vi "ExportToXMI.vi"(0 "reference":refnum<class "ClassDiagramGraph.lvclass">, 1 "nodeInfo":T2, 2 "edgeInfo":T1, 3 "DiagramData":string, 5 "error in (no error)":errorcluster) -> (14 "reference out":refnum<class "ClassDiagramGraph.lvclass">, 16 "XMIText":string, 19 "error out":errorcluster)   [LabVIEW 2016, in "ClassDiagramGraph.lvclass"]
uses:
  <resource>/Framework/Providers/Open_GDS/UML/ClassDiagramGraph_class/ClassDiagramGraph.lvclass
  C:/Program Files (x86)/National Instruments/LabVIEW 2016/resource/Framework/Providers/Open_GDS/UML/Graph_class/Graph.lvclass
  <resource>/Framework/Providers/Open_GDS/ClassProviders/Common/CommonVIs/CommonVIs_ClassNamePathType.ctl
  <resource>/Framework/Providers/Open_GDS/ClassProviders/Common/CommonVIs/CommonVIs_AttributeType.ctl
  <resource>/Framework/Providers/Open_GDS/ClassProviders/Common/CommonVIs/CommonVIs_AttributeDataType.ctl
  <resource>/Framework/Providers/Open_GDS/ClassProviders/Common/String/GDSString_AccessScopeModifierType.ctl
  <resource>/Framework/Providers/Open_GDS/UML/ClassRelationshipEdge_class/private/AssociationType.ctl
  <resource>/Framework/Providers/Open_GDS/UML/General/Point/Point Point2D.ctl
  <resource>/Framework/Providers/Open_GDS/UML/LineStyle_class/LineStyleType.ctl
  <resource>/Framework/Providers/Open_GDS/UML/ArrowHead_class/ArrowHeadType.ctl
  <resource>/Framework/Providers/Open_GDS/UML/PackageNode_class/PackageNode.lvclass
  <resource>/Framework/Providers/Open_GDS/UML/ClassNode_class/ClassNode.lvclass
  <resource>/Framework/Providers/Open_GDS/UML/ArrowHead_class/ArrowHead.lvclass
  <resource>/Framework/Providers/Open_GDS/UML/ClassRelationshipEdge_class/ClassRelationshipEdge.lvclass
  <resource>/Framework/Providers/Open_GDS/UML/LineStyle_class/LineStyle.lvclass
  <resource>/Framework/Providers/Open_GDS/UML/Graph_class/Graph.lvclass
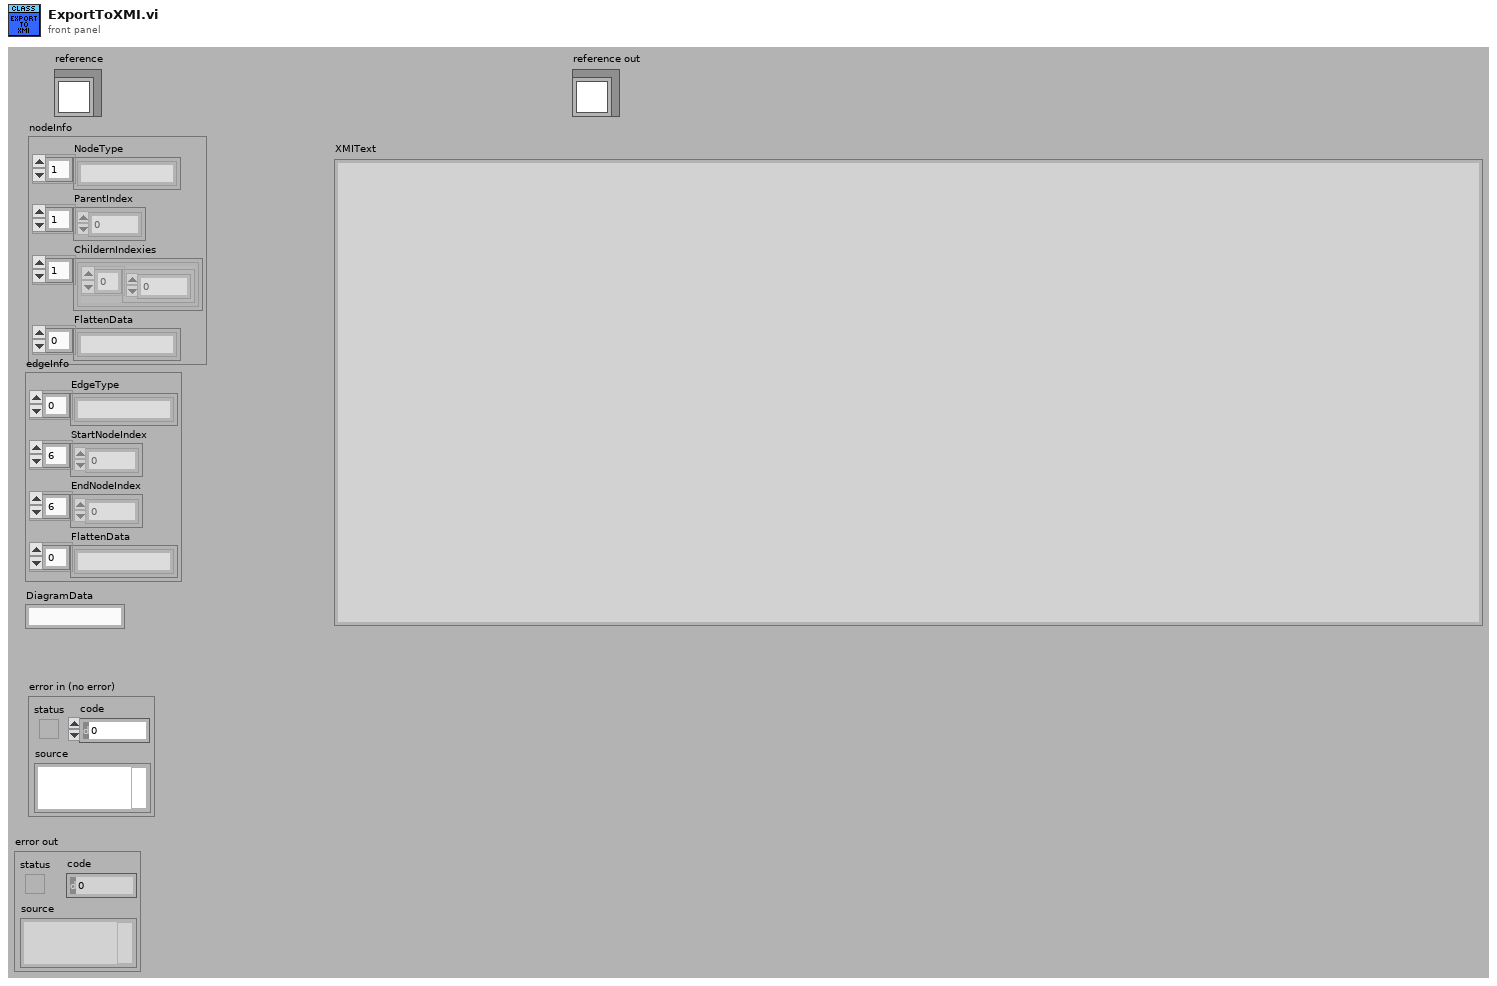
[diagram p1: front panel]
types:
  T1 = cluster{"EdgeType":string[], "StartNodeIndex":i32[], "EndNodeIndex":i32[], "FlattenData":string[]}
  T2 = cluster{"NodeType":string[], "ParentIndex":i32[], "ChildernIndexies":cluster{i32[]}[], "FlattenData":string[]}
  T3 = typedef "CommonVIs_ClassNamePathType.ctl" = cluster{"ClassNamn":string, "ClassPath":path, "InterfaceClass":bool}
  T4 = typedef "CommonVIs_AttributeType.ctl" = cluster{"Name":string, "DataType":T5, "ArrayDim":i32, "CtrlPath":path, "DataTypeString":string, "AccessScope":T6, "InitialData":variant}
  T5 = typedef "CommonVIs_AttributeDataType.ctl" = enum16{"UINT8", "INT8", "UINT16", "INT16", "UINT32", "INT32", "UINT64", "INT64", "SGL", "DBL", "EXT", "CSG", "CDB", "CXT", "TimeStamp", "STRING", "PATH", "BOOL", "ENUM", "RefNum", "VIRefNum", "LabVIEW Class", "Cluster", "Variant", "TypeDef", "Waveform", "LabVIEW Object", "Other", "void"}
  T6 = typedef "GDSString_AccessScopeModifierType.ctl" = enum16{"public", "private", "protected", "internal"}
  T7 = typedef "ClassRelationshipEdge.lvclass/AssociationType.ctl" = u16
  T8 = cluster{"NodeNames":string[], "Attributes":cluster{"attributes":string[]}[], "Methods":cluster{"attributes":string[]}[], "StereoType":string[], "ClassInfo":T3[], "ClassAttributes":cluster{"Attributes":T4[]}[], "RelationShipTypes":T7[], "DataTypes":T5[], "NodeTypes":enum16{"Class", "NotSpecified", "Package", "Note", "Interface"}[], "Text":string, "NodeRelationships":cluster{cluster{"index of element":i32, "RelationType":T7}[]}[], "Ass":cluster{string, i32, "index of element":i32}[]}
  T9 = typedef "Point Point2D.ctl" = cluster{"x":dbl, "y":dbl}
  T10 = cluster{"Attributes":cluster{"Base class":cluster{"Base class":cluster{"Base class":cluster{"start":refnum<k1>, "end":refnum<k1>}}, "lineStyle":refnum<k1>, "startArrowHead":refnum<k1>, "endArrowHead":refnum<k1>, "startLabel":string, "midLabel":string, "endLabel":string, "MidLabelOffset":T9, "SplitWire":bool}, "bentStyleRef":refnum<k1>, "startConnectionOffset":cluster{"x":i32, "y":i32}, "endConnectionOffset":cluster{"x":i32, "y":i32}, "MidLineOffset":cluster{"x":i32, "y":i32}, "DepClass":cluster{"ThisVIs/Ctls":path[], "Dependent_VIs/Ctls":path[]}}, string, string, string, string}
  T11 = typedef "ArrowHead.lvclass/ArrowHeadType.ctl" = enum16{"NONE", "TRIANGLE", "BLACK_TRIANGLE", "V", "HALF_V", "DIAMOND", "BLACK_DIAMOND"}
  T12 = typedef "LineStyle.lvclass/LineStyleType.ctl" = enum16{"SOLID", "DOTTED"}
  T13 = cluster{"index of element":i32, "RelationType":T7}[]
  T14 = enum16{"Class", "NotSpecified", "Package", "Note", "Interface"}
  T15 = typedef "Graph.lvclass/ObjectAttributes.ctl" = cluster{"nodes":refnum<class "AbstractNode.lvclass">[], "edges":refnum<class "AbstractEdge.lvclass">[], "nodesToBeRemoved":refnum<class "AbstractNode.lvclass">[], "edgesToBeRemoved":refnum<class "AbstractEdge.lvclass">[], "needsLayout":bool, "LayoutNodes":refnum<class "AbstractNode.lvclass">[]}
  T16 = cluster{"index of element":i32, "RelationType":T7}
  T17 = cluster{cluster{"index of element":i32, "RelationType":T7}[]}
  T18 = enum16{"Class", "NotSpecified", "Package", "Note", "Interface"}[]
  T19 = cluster{cluster{"index of element":i32, "RelationType":T7}[]}[]
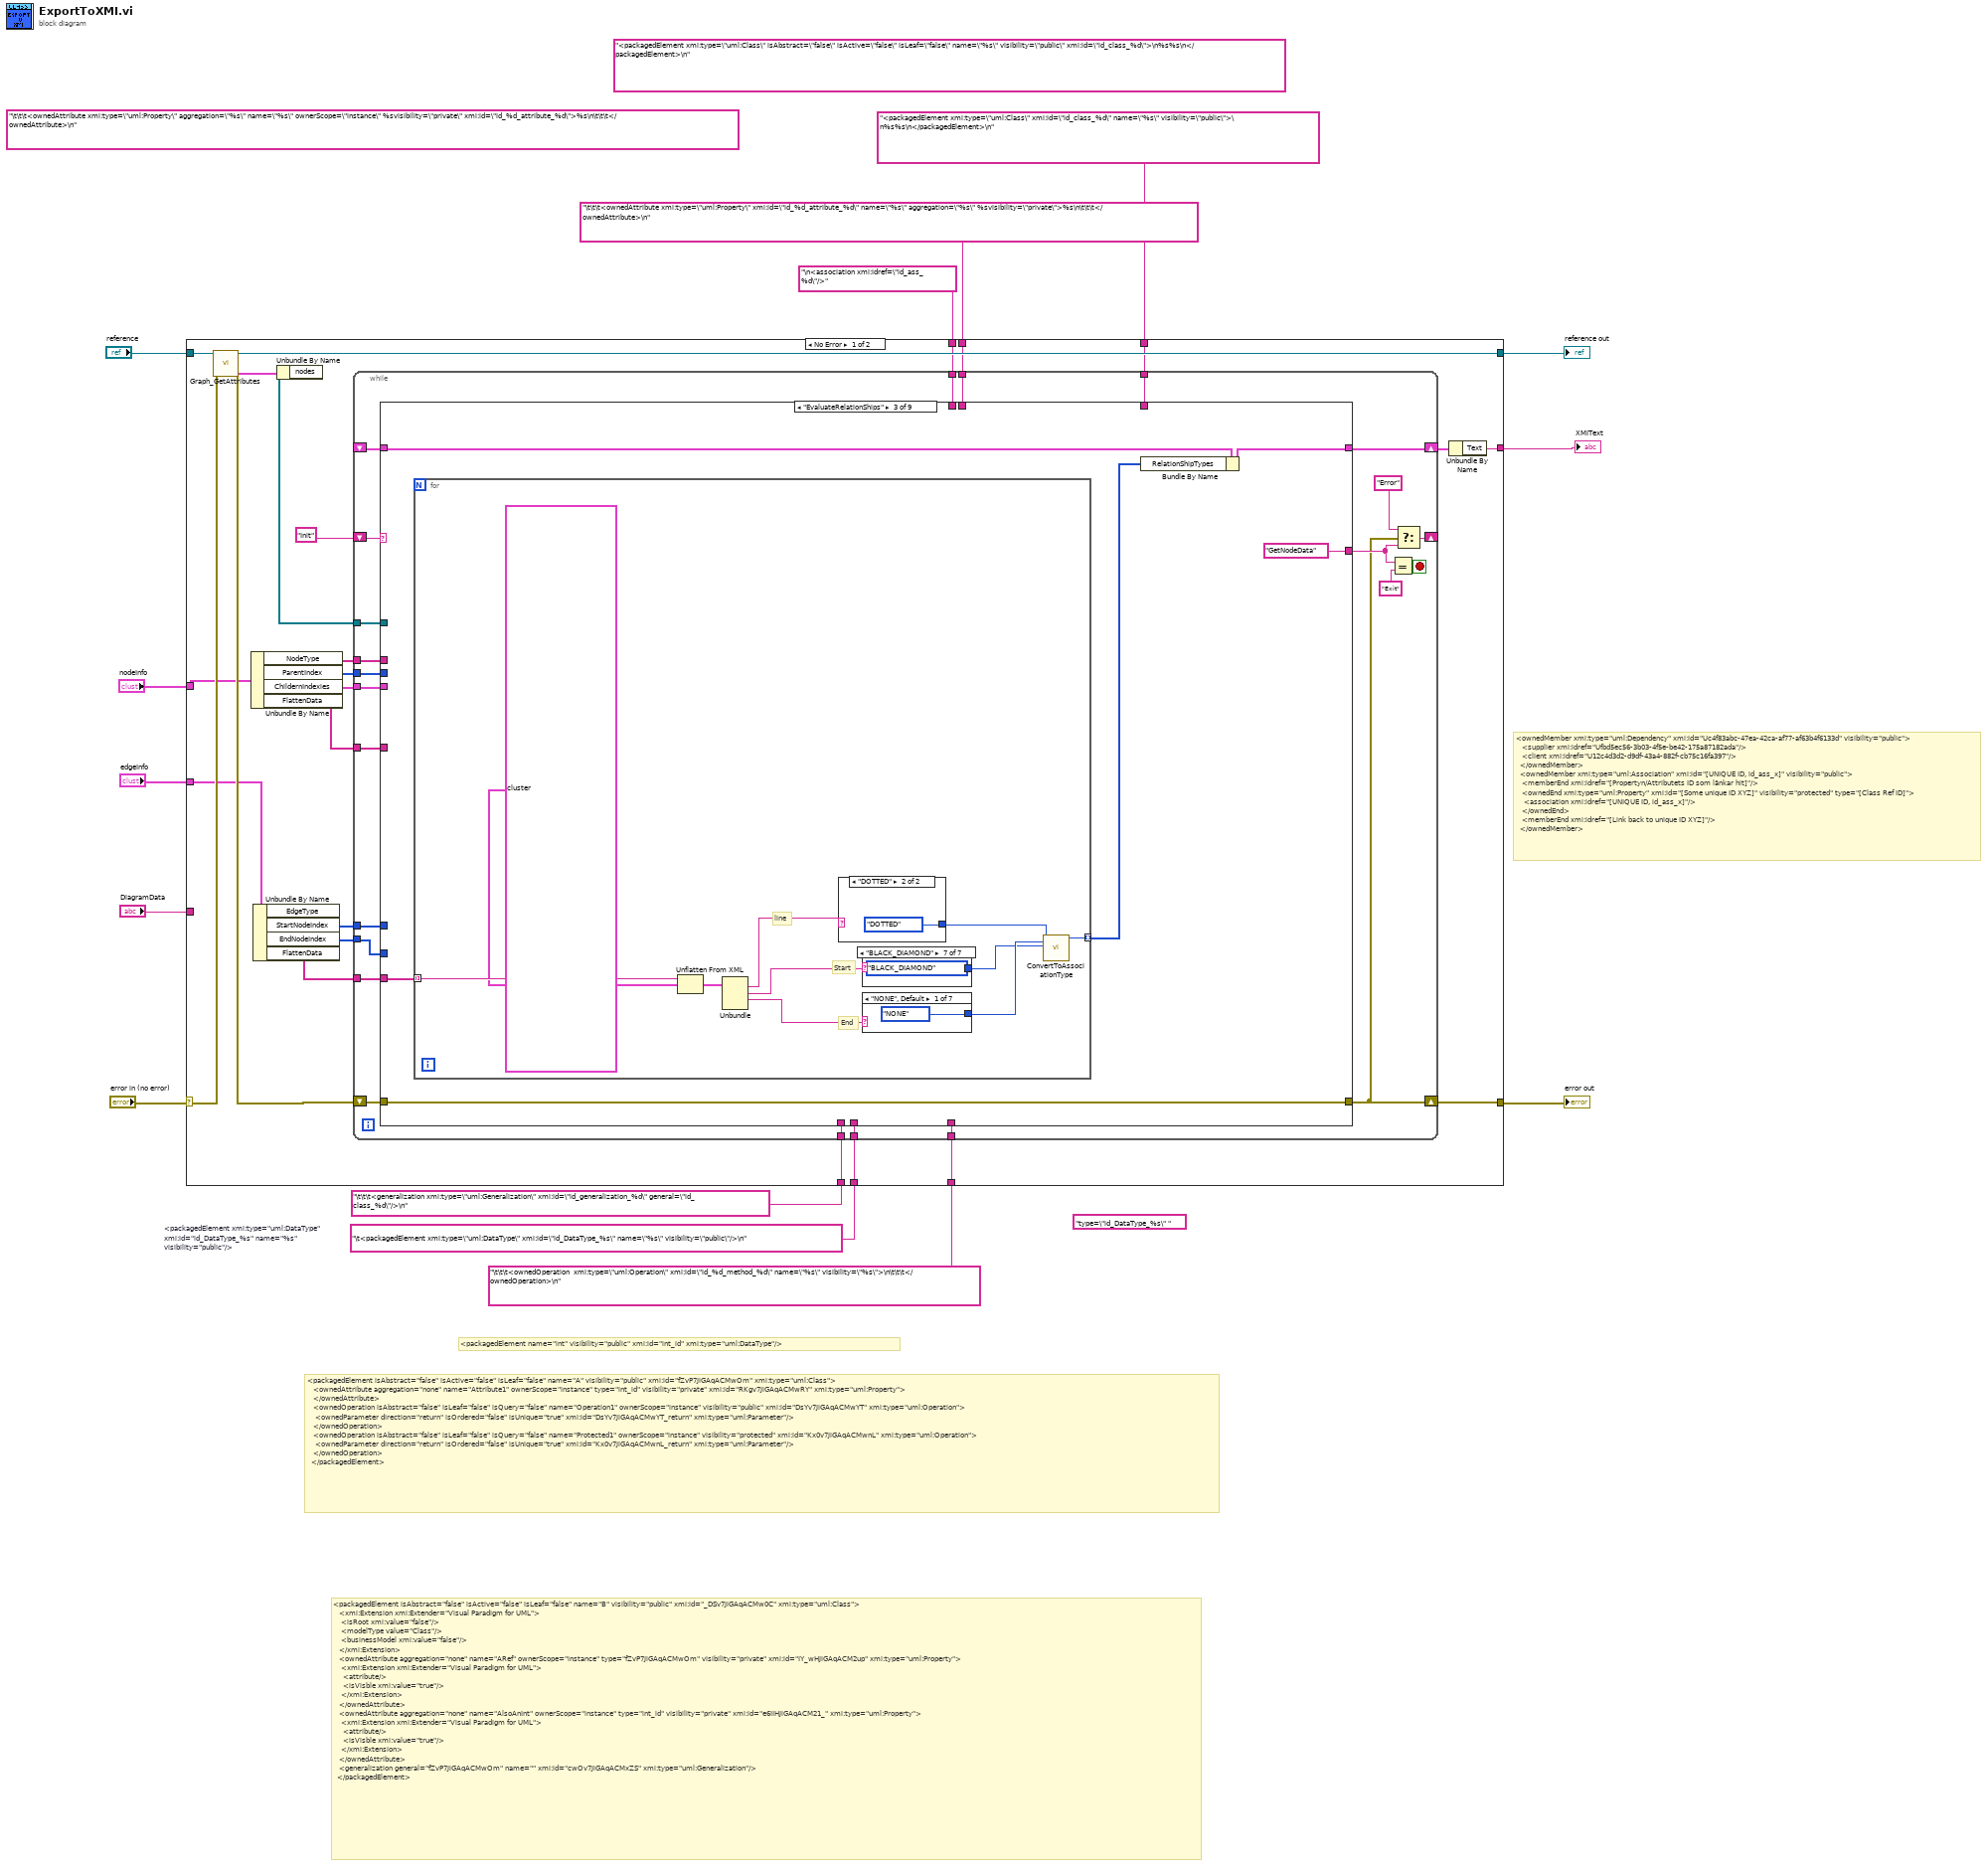
[diagram p0: block diagram]
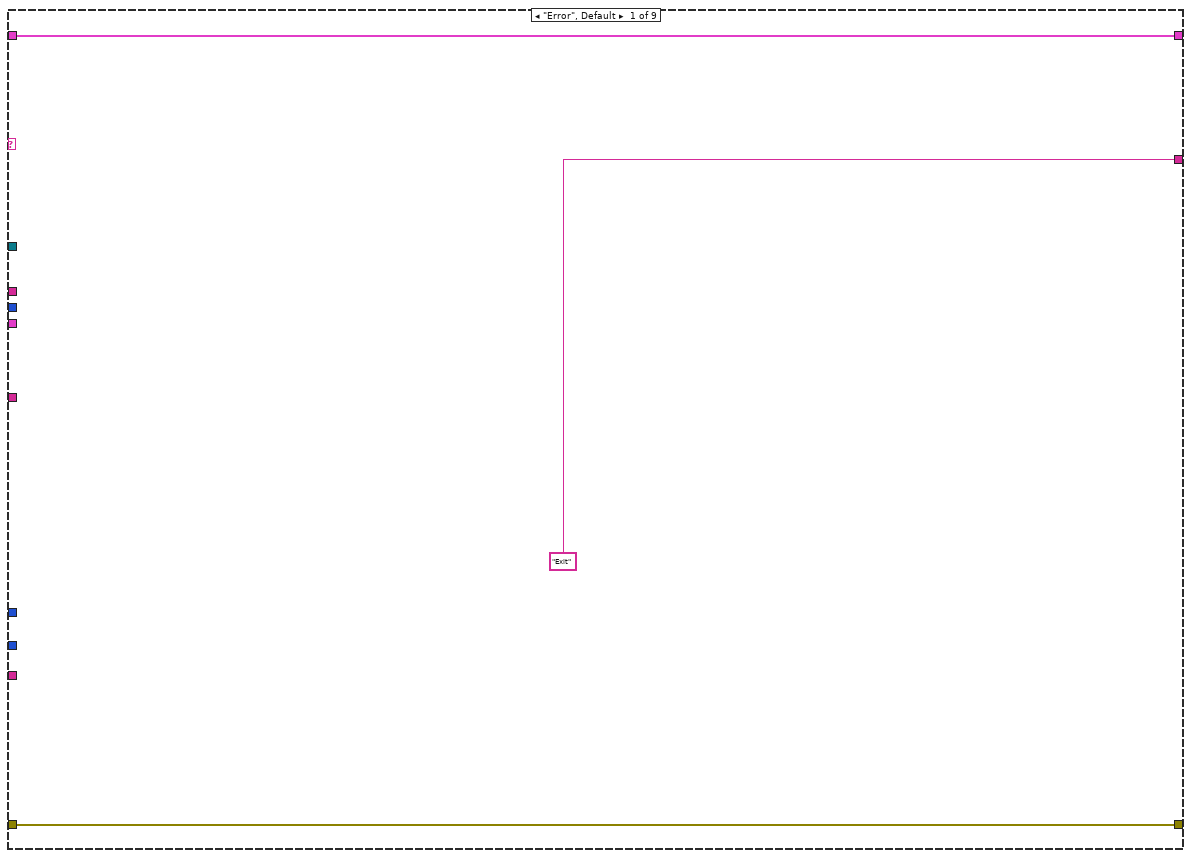
[diagram p2: hidden frame]
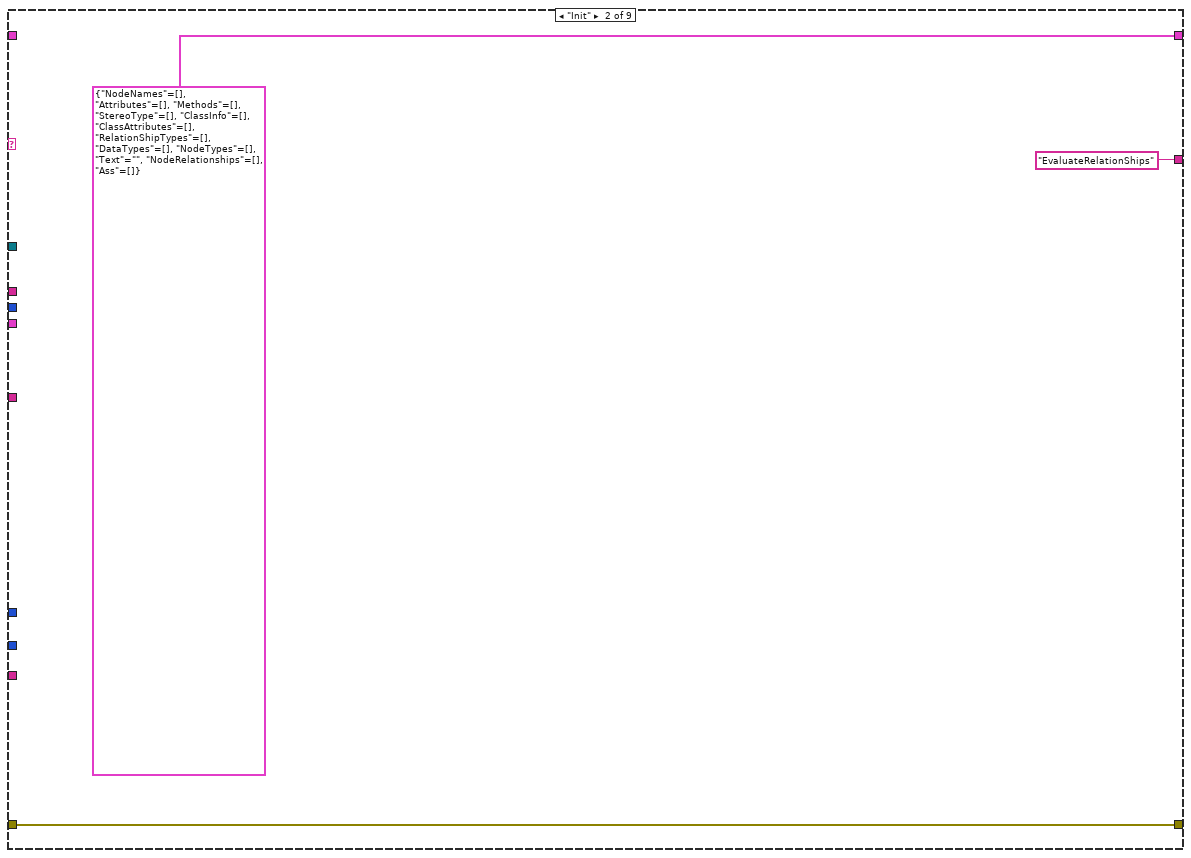
[diagram p3: hidden frame]
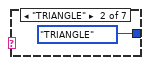
[diagram p4: hidden frame]
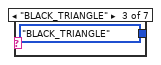
[diagram p5: hidden frame]
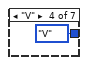
[diagram p6: hidden frame]
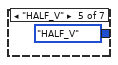
[diagram p7: hidden frame]
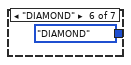
[diagram p8: hidden frame]
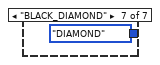
[diagram p9: hidden frame]
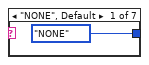
[diagram p10: hidden frame]
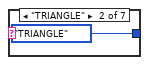
[diagram p11: hidden frame]
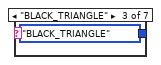
[diagram p12: hidden frame]
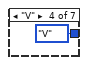
[diagram p13: hidden frame]
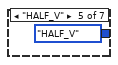
[diagram p14: hidden frame]
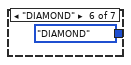
[diagram p15: hidden frame]
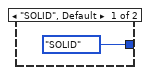
[diagram p16: hidden frame]
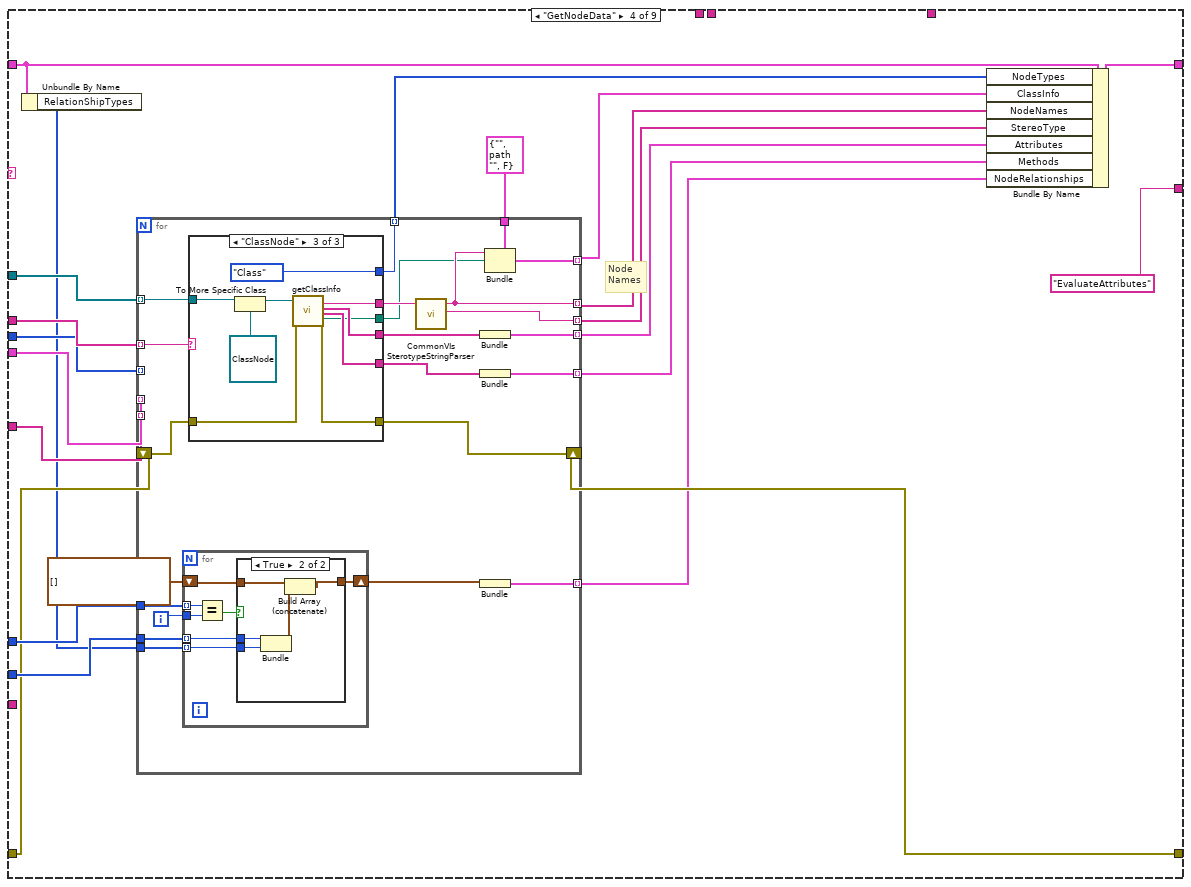
[diagram p17: hidden frame]
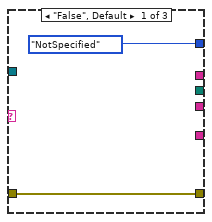
[diagram p19: hidden frame]
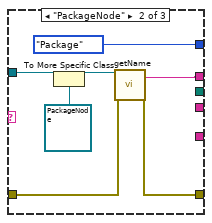
[diagram p20: hidden frame]
diagram:
  (unwired) "\t\t\t<ownedAttribute xmi:type=\"uml:Property\" aggregation=\"%s\" name=\"%s\" ownerScope=\"instance\" %svisibility=\"private\" xmi:id=\"id_%d_attribute_%d\">%s\n\t\t\t</ownedAttribute>\n" ("format string")
  (unwired) "<packagedElement xmi:type=\"uml:Class\" isAbstract=\"false\" isActive=\"false\" isLeaf=\"false\" name=\"%s\" visibility=\"public\" xmi:id=\"id_class_%d\">\n%s%s\n</packagedElement>\n" ("format string")
  (unwired) "type=\"id_DataType_%s\" " ("input 1")
  w4 = "\t<packagedElement xmi:type=\"uml:DataType\" xmi:id=\"id_DataType_%s\" name=\"%s\" visibility=\"public\"/>\n"  # <packagedElement xmi:type="uml:DataType" xmi:id="id_DataType_%s" name="%s" visibility="public"/>
  # "<ownedMember xmi:type=\"uml:Dependency\" xmi:id=\"Uc4f83abc-47ea-42ca-af77-af63b4f6133d\" visibility=\"public\">\n\t\t\t<supplier xmi:idref=\"Ufbd5ec56-3b03-4f5e-be42-175a87182ada\"/>\n\t\t\t<client xmi:idref=\"U12c4d3d2-d9df-43a4-882f-cb75c16fa397\"/>\n\t\t</ownedMember>\n\t\t<ownedMember xmi:type=\"uml:Association\" xmi:id=\"[UNIQUE ID, id_ass_x]\" visibility=\"public\">\n\t\t\t<memberEnd xmi:idref=\"[Propertyn/Attributets ID som länkar hit]\"/>\n\t\t\t<ownedEnd xmi:type=\"uml:Property\" xmi:id=\"[Some unique ID XYZ]\" visibility=\"protected\" type=\"[Class Ref ID]\">\n\t\t\t\t<association xmi:idref=\"[UNIQUE ID, id_ass_x]\"/>\n\t\t\t</ownedEnd>\n\t\t\t<memberEnd xmi:idref=\"[Link back to unique ID XYZ]\"/>\n\t\t</ownedMember>"
  # "<packagedElement isAbstract=\"false\" isActive=\"false\" isLeaf=\"false\" name=\"B\" visibility=\"public\" xmi:id=\"_DSv7JiGAqACMw0C\" xmi:type=\"uml:Class\">\n\t\t\t<xmi:Extension xmi:Extender=\"Visual Paradigm for UML\">\n\t\t\t\t<isRoot xmi:value=\"false\"/>\n\t\t\t\t<modelType value=\"Class\"/>\n\t\t\t\t<businessModel xmi:value=\"false\"/>\n\t\t\t</xmi:Extension>\n\t\t\t<ownedAttribute aggregation=\"none\" name=\"ARef\" ownerScope=\"instance\" type=\"fZvP7JiGAqACMwOm\" visibility=\"private\" xmi:id=\"IY_wHJiGAqACM2up\" xmi:type=\"uml:Property\">\n\t\t\t\t<xmi:Extension xmi:Extender=\"Visual Paradigm for UML\">\n\t\t\t\t\t<attribute/>\n\t\t\t\t\t<isVisble xmi:value=\"true\"/>\n\t\t\t\t</xmi:Extension>\n\t\t\t</ownedAttribute>\n\t\t\t<ownedAttribute aggregation=\"none\" name=\"AlsoAnInt\" ownerScope=\"instance\" type=\"int_id\" visibility=\"private\" xmi:id=\"e6IIHJiGAqACM21_\" xmi:type=\"uml:Property\">\n\t\t\t\t<xmi:Extension xmi:Extender=\"Visual Paradigm for UML\">\n\t\t\t\t\t<attribute/>\n\t\t\t\t\t<isVisble xmi:value=\"true\"/>\n\t\t\t\t</xmi:Extension>\n\t\t\t</ownedAttribute>\n\t\t\t<generalization general=\"fZvP7JiGAqACMwOm\" name=\"\" xmi:id=\"cwOv7JiGAqACMxZS\" xmi:type=\"uml:Generalization\"/>\n\t\t</packagedElement>"
  # "<packagedElement isAbstract=\"false\" isActive=\"false\" isLeaf=\"false\" name=\"A\" visibility=\"public\" xmi:id=\"fZvP7JiGAqACMwOm\" xmi:type=\"uml:Class\">\n\t\t\t<ownedAttribute aggregation=\"none\" name=\"Attribute1\" ownerScope=\"instance\" type=\"int_id\" visibility=\"private\" xmi:id=\"RKgv7JiGAqACMwRY\" xmi:type=\"uml:Property\">\n\t\t\t</ownedAttribute>\n\t\t\t<ownedOperation isAbstract=\"false\" isLeaf=\"false\" isQuery=\"false\" name=\"Operation1\" ownerScope=\"instance\" visibility=\"public\" xmi:id=\"DsYv7JiGAqACMwYT\" xmi:type=\"uml:Operation\">\n\t\t\t\t<ownedParameter direction=\"return\" isOrdered=\"false\" isUnique=\"true\" xmi:id=\"DsYv7JiGAqACMwYT_return\" xmi:type=\"uml:Parameter\"/>\n\t\t\t</ownedOperation>\n\t\t\t<ownedOperation isAbstract=\"false\" isLeaf=\"false\" isQuery=\"false\" name=\"Protected1\" ownerScope=\"instance\" visibility=\"protected\" xmi:id=\"Kx0v7JiGAqACMwnL\" xmi:type=\"uml:Operation\">\n\t\t\t\t<ownedParameter direction=\"return\" isOrdered=\"false\" isUnique=\"true\" xmi:id=\"Kx0v7JiGAqACMwnL_return\" xmi:type=\"uml:Parameter\"/>\n\t\t\t</ownedOperation>\n\t\t</packagedElement>"
  # "<packagedElement name=\"int\" visibility=\"public\" xmi:id=\"int_id\" xmi:type=\"uml:DataType\"/>"
  n1 = case shown="No Error" "error in (no error)" {
    selector: "error in (no error)" -> [w37 w452]
    tunnel: "reference" -> [w39 w453]
    tunnel: [w28 w452] -> w13
    tunnel: [w38 w453] -> w12
    tunnel: "nodeInfo" -> [w33 _]
    tunnel: "edgeInfo" -> [w27 _]
    tunnel: "DiagramData" -> [_ _]
    tunnel: "<packagedElement xmi:type=\"uml:Class\" xmi:id=\"id_class_%d\" name=\"%s\" visibility=\"public\">\n%s%s\n</packagedElement>\n" ("format string") -> [w23 _]
    tunnel: "\t\t\t<ownedAttribute xmi:type=\"uml:Property\" xmi:id=\"id_%d_attribute_%d\" name=\"%s\" aggregation=\"%s\" %svisibility=\"private\">%s\n\t\t\t</ownedAttribute>\n" ("format string") -> [w22 _]
    tunnel: "\t\t\t<ownedOperation  xmi:type=\"uml:Operation\" xmi:id=\"id_%d_method_%d\" name=\"%s\" visibility=\"%s\">\n\t\t\t</ownedOperation>\n" -> [w21 _]
    tunnel: w4 -> [w20 _]
    tunnel: [w18 _] -> w3
    tunnel: "\t\t\t<generalization xmi:type=\"uml:Generalization\" xmi:id=\"id_generalization_%d\" general=\"id_class_%d\"/>\n" ("input 1") -> [w17 _]
    tunnel: "\n<association xmi:idref=\"id_ass_%d\"/>" ("input 1") -> [w16 _]
    frame No Error {
      n2 = call <resource>:"Graph_GetAttributes.vi"("reference in"=w39, "error in (no error)"=w37) -> ("reference out"=w38:refnum<class "ClassDiagramGraph.lvclass">, "Data"=w15:T15, "error out"=w35:errorcluster)  [unwired: 14 in, 1 out]
      n3 = Unbundle By Name(w33) -> ("NodeType"=w32:string[], "ParentIndex"=w31:i32[], "ChildernIndexies"=w30:cluster{i32[]}[], "FlattenData"=w29:string[])
      n4 = Unbundle By Name(w27) -> ("StartNodeIndex"=w26:i32[], "EndNodeIndex"=w25:i32[], "FlattenData"=w24:string[])  [unwired: 1 out]
      n5 = Unbundle By Name(w15) -> ("nodes"=w34:refnum<class "AbstractNode.lvclass">[])
      n6 = while {
        shift-right: [w57] -> w28
        shift-left: w35 -> [w63]
        shift-right: [w61] -> _
        shift-left: "Init" -> [w62]
        shift-right: [w56] -> w19
        shift-left: _ -> [w55]
        tunnel: w34 -> [w54]
        tunnel: w32 -> [w53]
        tunnel: w31 -> [w52]
        tunnel: w30 -> [w51]
        tunnel: w29 -> [w50]
        tunnel: w26 -> [w49]
        tunnel: w25 -> [w48]
        tunnel: w24 -> [w47]
        tunnel: w23 -> [w46]
        tunnel: w22 -> [w45]
        tunnel: w21 -> [w44]
        tunnel: w20 -> [w43]
        tunnel: w17 -> [w42]
        tunnel: w16 -> [w41]
        stop <- w60 stop-if-true
        n7 = case shown="\"EvaluateRelationShips\"" w62 {
          tunnel: w63 -> [w66 w69 w72 w112 w179 w211 w381 w396 w416]
          tunnel: [w66 w69 w72 w111 w179 w211 w381 w396 w416] -> w57
          tunnel: ["Exit" "EvaluateRelationShips" "GetNodeData" "EvaluateAttributes" "XMI:CreateClasses" "CreateDataTypes" "CreateReferedAssociations" "CreateNormalAssociations" "Exit"] -> w58
          tunnel: [w64 T8 {"NodeNames"=[], "Attributes"=[], "Methods"=[], "StereoType"=[], "ClassInfo"=[], "ClassAttributes"=[], "RelationShipTypes"=[], "DataTypes"=[], "NodeTypes"=[], "Text"="", "NodeRelationships"=[], "Ass"=[]} w74 w116 w180 w218 w385 w399 w419] -> w56
          tunnel: w55 -> [w64 _ w75 w105 w182 w219 w386 w400 w410]
          tunnel: w54 -> [_ _ _ w121 _ _ _ _ _]
          tunnel: w53 -> [_ _ _ w120 _ _ _ _ _]
          tunnel: w52 -> [_ _ _ w119 _ _ _ _ _]
          tunnel: w51 -> [_ _ _ w118 _ _ _ _ _]
          tunnel: w50 -> [_ _ _ w117 _ _ _ _ _]
          tunnel: w49 -> [_ _ _ w114 _ _ _ _ _]
          tunnel: w48 -> [_ _ _ w113 _ _ _ _ _]
          tunnel: w47 -> [_ _ w73 _ _ _ _ _ _]
          tunnel: w46 -> [_ _ _ _ _ w221 w387 w401 w420]
          tunnel: w45 -> [_ _ _ _ _ w216 w383 w397 w417]
          tunnel: w44 -> [_ _ _ _ _ w212 w382 _ _]
          tunnel: w43 -> [_ _ _ _ _ _ w379 _ _]
          tunnel: w42 -> [_ _ _ _ _ w209 _ _ _]
          tunnel: w41 -> [_ _ _ _ _ w207 _ _ _]
          frame "Error", Default {
          }
          frame "Init" {
          }
          frame "EvaluateRelationShips" {
            n8 = for {
              tunnel: w73 -> [w85] mode=indexing
              tunnel: [w77] -> w71 mode=indexing
              # "End"
              # "Start"
              # "line"
              n9 = Unflatten From XML(xml string=w85, type=T10 {"Attributes"={"Base class"={"Base class"={"Base class"={"start"=refnum, "end"=refnum}}, "lineStyle"=refnum, "startArrowHead"=refnum, "endArrowHead"=refnum, "startLabel"="", "midLabel"="", "endLabel"="", "MidLabelOffset"={"x"=0.0, "y"=0.0}, "SplitWire"=FALSE}, "bentStyleRef"=refnum, "startConnectionOffset"={"x"=0, "y"=0}, "endConnectionOffset"={"x"=0, "y"=0}, "MidLineOffset"={"x"=0, "y"=0}, "DepClass"={"ThisVIs/Ctls"=[], "Dependent_VIs/Ctls"=[]}}, "", "", "", ""} ("output cluster")) -> (value=w84:T10)  [unwired: 1 in, 1 out]
              n10 = Unbundle(w84) -> (w83:string, w82:string, w81:string)  [unwired: 2 out]
              n11 = case shown="\"DOTTED\"" w83 {
                tunnel: [LineStyleType."SOLID" ("lineStyle") LineStyleType."DOTTED" ("lineStyle")] -> w80
                frame "SOLID", Default {
                }
                frame "DOTTED" {
                }
              }
              n12 = case shown="\"BLACK_DIAMOND\"" w82 {
                tunnel: [ArrowHeadType."NONE" ("arrowHead") ArrowHeadType."TRIANGLE" ("arrowHead") ArrowHeadType."BLACK_TRIANGLE" ("arrowHead") ArrowHeadType."V" ("arrowHead") ArrowHeadType."HALF_V" ("arrowHead") ArrowHeadType."DIAMOND" ("arrowHead") ArrowHeadType."BLACK_DIAMOND" ("arrowHead")] -> w78
                frame "NONE", Default {
                }
                frame "TRIANGLE" {
                }
                frame "BLACK_TRIANGLE" {
                }
                frame "V" {
                }
                frame "HALF_V" {
                }
                frame "DIAMOND" {
                }
                frame "BLACK_DIAMOND" {
                }
              }
              n13 = case shown="\"NONE\", Default" w81 {
                tunnel: [ArrowHeadType."NONE" ("arrowHead") ArrowHeadType."TRIANGLE" ("arrowHead") ArrowHeadType."BLACK_TRIANGLE" ("arrowHead") ArrowHeadType."V" ("arrowHead") ArrowHeadType."HALF_V" ("arrowHead") ArrowHeadType."DIAMOND" ("arrowHead") ArrowHeadType."DIAMOND" ("arrowHead")] -> w79
                frame "NONE", Default {
                }
                frame "TRIANGLE" {
                }
                frame "BLACK_TRIANGLE" {
                }
                frame "V" {
                }
                frame "HALF_V" {
                }
                frame "DIAMOND" {
                }
                frame "BLACK_DIAMOND" {
                }
              }
              n14 = call <resource>:"ConvertToAssociationType.vi"("lineStyle"=w80, "EndArrowHead"=w79, "StartArrowHead"=w78) -> ("RelationType"=w77:T7)  [unwired: 16 out]
            }
            n15 = Bundle By Name(cluster=w75, "RelationShipTypes"=w71) -> (w74:T8)
          }
          frame "GetNodeData" {
            # "Node\nNames"
            n16 = Unbundle By Name(w105) -> ("RelationShipTypes"=w104:T7[])
            n17 = for {
              tunnel: w121 -> [w142] mode=indexing
              tunnel: w120 -> [w143] mode=indexing
              tunnel: w119 -> [_] mode=indexing
              tunnel: w118 -> [_] mode=indexing
              tunnel: w117 -> [_] mode=indexing
              shift-right: [w140] -> w111
              shift-left: w112 -> [w141]
              tunnel: [w128] -> w115 mode=indexing
              tunnel: w114 -> [w139]
              tunnel: w113 -> [w137]
              tunnel: [w135] -> w103 mode=indexing
              tunnel: [w133] -> w110 mode=indexing
              tunnel: [w131] -> w109 mode=indexing
              tunnel: [w130] -> w108 mode=indexing
              tunnel: T3 {"ClassNamn"="", "ClassPath"=path "", "InterfaceClass"=FALSE} ("Cluster") -> [w129]
              tunnel: [w126] -> w107 mode=indexing
              tunnel: [w125] -> w106 mode=indexing
              tunnel: w104 -> [w124]
              i -> [w138]
              n18 = for {
                tunnel: w139 -> [w150] mode=indexing
                tunnel: w138 -> [w149]
                shift-right: [w145] -> w136
                shift-left: T13 [] -> [w147]
                tunnel: w137 -> [w146] mode=indexing
                tunnel: w124 -> [w144] mode=indexing
                n19 = Equal?(x=w150, y=w149) -> (x = y?=w148:bool)
                n20 = case shown="True" w148 {
                  tunnel: w147 -> [w151 w156]
                  tunnel: w146 -> [_ w153]
                  tunnel: [w151 w155] -> w145
                  tunnel: w144 -> [_ w154]
                  frame False {
                  }
                  frame True {
                    n21 = Bundle("index of element"=w153, "RelationType"=w154) -> (w152:T16)  [unwired: 1 out]
                    n22 = Build Array (concatenate)(w156, w152) -> (w155:T13)
                  }
                }
              }
              n23 = case shown="\"ClassNode\"" w143 {
                tunnel: w142 -> [_ w161 w168]
                tunnel: w141 -> [w158 w165 w175]
                tunnel: [w158 w164 w174] -> w140
                tunnel: [_ w163 w173] -> w128
                tunnel: [_ _ w172] -> w134
                tunnel: [_ _ w171] -> w132
                tunnel: [_ _ w170] -> w127
                tunnel: [T14."NotSpecified" T14."Package" T14."Class"] -> w125
                frame "False", Default {
                }
                frame "PackageNode" {
                  n24 = To More Specific Class(target class=refnum<class "PackageNode.lvclass"> refnum ("reference"), reference=w161) -> (specific class reference=w160:refnum<class "PackageNode.lvclass">)  [unwired: 1 in, 1 out]
                  n25 = call-dynamic "getName.vi"("reference"=w160, "error in (no error)"=w165) -> ("name"=w163:string, "error out"=w164:errorcluster)  [unwired: 15 in, 1 out]
                }
                frame "ClassNode" {
                  n26 = To More Specific Class(target class=refnum<class "ClassNode.lvclass"> refnum ("reference"), reference=w168) -> (specific class reference=w167:refnum<class "ClassNode.lvclass">)  [unwired: 1 in, 1 out]
                  n27 = call-dynamic "getClassInfo.vi"("reference"=w167, "error in (no error)"=w175) -> ("className"=w173:string, "attributes"=w172:string[], "methods"=w171:string[], "ClassPath"=w170:path, "error out"=w174:errorcluster)  [unwired: 8 in, 5 out]
                }
              }
              n28 = call <resource>:"CommonVIs SterotypeStringParser.vi"("SterotypeStringIn"=w128) -> ("Sterotype"=w130:string)  [unwired: 18 out]
              n29 = Bundle("attributes"=w134) -> (w133:cluster{"attributes":string[]})  [unwired: 1 in]
              n30 = Bundle("methods"=w132) -> (w131:cluster{"methods":string[]})  [unwired: 1 in]
              n31 = Bundle(w136) -> (w135:T17)  [unwired: 1 in]
              n32 = Bundle(cluster=w129, "ClassNamn"=w128, "ClassPath"=w127) -> (w126:T3)  [unwired: 1 out]
            }
            n33 = Bundle By Name(cluster=w105, "NodeTypes"=w106, "ClassInfo"=w107, "NodeNames"=w115, "StereoType"=w108, "Attributes"=w110, "Methods"=w109, "NodeRelationships"=w103) -> (w116:T8)
          }
          frame "EvaluateAttributes" {
            w178 = T5[] [] items=["UINT8", "INT8", "UINT16", "INT16", "UINT32", "INT32", "UINT64", "INT64", "SGL", "DBL", "EXT", "CSG", "CDB", "CXT", "TimeStamp", "STRING", "PATH", "BOOL", "ENUM", "RefNum", "VIRefNum", "LabVIEW Class", "Cluster", "Variant", "TypeDef", "Waveform", "LabVIEW Object", "Other", "void"]
            n34 = Unbundle By Name(w182) -> ("Attributes"=w184:cluster{"attributes":string[]}[], "ClassInfo"=w183:T3[])
            n35 = for {
              tunnel: w184 -> [w191] mode=indexing
              tunnel: w183 -> [w189]
              tunnel: [w188] -> w181 mode=indexing
              shift-right: [w185] -> w177
              shift-left: w178 -> [w186]
              n36 = Unbundle(w191) -> ("attributes"=w190:string[])
              n37 = call <resource>:"ReversedEngineering_AttributeToDataType.vi"("ClassInfo"=w189, "Array"=w190) -> ("Attributes"=w187:T4[])
              n38 = for {
                tunnel: w187 -> [w196] mode=indexing
                shift-right: [w192] -> w185
                shift-left: w186 -> [w194]
                n39 = Unbundle By Name(w196) -> ("DataType"=w193:T5)
                n40 = Search 1D Array(1D array=w194, element=w193) -> (index of element=w195:i32)  [unwired: 1 out]
                n41 = case shown="-1" w195 {
                  tunnel: w194 -> [w197 w200]
                  tunnel: w193 -> [_ w198]
                  tunnel: [w197 w199] -> w192
                  frame 0, Default {
                  }
                  frame -1 {
                    n42 = case shown="\"Other\"" w198 {
                      selector: w198 -> [_ w202]
                      tunnel: w200 -> [w201 w204]
                      tunnel: [w201 w203] -> w199
                      frame "Other" {
                      }
                      frame Default {
                        n43 = Build Array (concatenate)(w204, w202) -> (w203:T5[])
                      }
                    }
                  }
                }
              }
              n44 = Bundle("Attributes"=w187) -> (w188:cluster{"Attributes":T4[]})  [unwired: 1 in]
            }
            n45 = Bundle By Name(cluster=w182, "ClassAttributes"=w181, "DataTypes"=w177) -> (w180:T8)
          }
          frame "XMI:CreateClasses" {
            # "aggregation=\"shared\""
            # "If attribute is an agg add:\n\t\t\t\t<association xmi:idref=\"U6ef3b323-399f-4cbb-b68b-93f0c12d382b\"/>"
            n46 = Unbundle By Name(w219) -> ("NodeTypes"=w222:T18, "NodeNames"=w208:string[], "ClassAttributes"=w214:cluster{"Attributes":T4[]}[], "Methods"=w213:cluster{"attributes":string[]}[], "NodeRelationships"=w210:T19)
            n47 = for {
              tunnel: w222 -> [w238] mode=indexing
              shift-right: [w235] -> w217
              shift-left: "" -> [w236]
              tunnel: w221 -> [w237]
              tunnel: w208 -> [w233] mode=indexing
              tunnel: w216 -> [w232]
              tunnel: w214 -> [w231] mode=indexing
              tunnel: w213 -> [w230] mode=indexing
              tunnel: w212 -> [w229]
              tunnel: w210 -> [w228] mode=indexing
              tunnel: w209 -> [w227]
              tunnel: w208 -> [w226]
              shift-right: [w223] -> w205
              shift-left: cluster{string, i32, "index of element":i32}[] [] -> [w225]
              tunnel: w207 -> [w224]
              i -> [w234]
              n48 = case shown="\"Class\"" w238 {
                tunnel: w237 -> [w267 _]
                tunnel: w236 -> [w266 w375]
                tunnel: [w265 w375] -> w235
                tunnel: w234 -> [w239 _]
                tunnel: w233 -> [w264 _]
                tunnel: w232 -> [w263 _]
                tunnel: w231 -> [w261 _]
                tunnel: w230 -> [w259 _]
                tunnel: w229 -> [w257 _]
                tunnel: w228 -> [w252 _]
                tunnel: w227 -> [w246 _]
                tunnel: w226 -> [w245 _]
                tunnel: w225 -> [w242 w374]
                tunnel: w224 -> [w241 _]
                tunnel: [w240 w374] -> w223
                frame "Class" {
                  (unwired) "Aggregations" ("input 1")
                  w249 = T7 1 items=["Depenency", "Inheritance", "Interface Implementation", "Association", "Aggregation", "Composite Aggregation"] ("element")
                  n49 = Unbundle(w261) -> ("Attributes"=w260:T4[])
                  n50 = Unbundle(w252) -> (w250:T13)
                  n51 = Unbundle(w259) -> ("attributes"=w258:string[])
                  n52 = for {
                    tunnel: w250 -> [w365] mode=indexing
                    tunnel: [w364] -> w243 mode=indexing
                    tunnel: [w363] -> w244 mode=indexing
                    n53 = Unbundle(w365) -> ("index of element"=w363:i32, "RelationType"=w364:T7)
                  }
                  n54 = for {
                    tunnel: w263 -> [w293]
                    shift-right: [w290] -> w253
                    shift-left: "" -> [w275]
                    tunnel: w260 -> [w292] mode=indexing
                    tunnel: w239 -> [w272]
                    tunnel: w245 -> [w289]
                    tunnel: w244 -> [w287]
                    tunnel: w243 -> [w285]
                    shift-right: [w281] -> w240
                    shift-left: w242 -> [w282]
                    tunnel: w241 -> [w280]
                    tunnel: w239 -> [w268]
                    i -> [w269]
                    n55 = Unbundle By Name(w292) -> ("Name"=w271:string, "DataType"=w288:T5, "DataTypeString"=w273:string)
                    n56 = Search 1D Array(1D array=w289, element=w273) -> (index of element=w286:i32)  [unwired: 1 out]
                    n57 = Search 1D Array(1D array=w287, element=w286) -> (index of element=w274:i32)  [unwired: 1 out]
                    n58 = Index Array(array=w285, index=w274) -> (element=w284:T7)
                    n59 = case shown="Default" w288 {
                      selector: w288 -> [w355 _]
                      tunnel: [w357 _] -> w279
                      tunnel: "type=\"id_DataType_%s\" " ("input 1") -> [w356 _]
                      frame Default {
                        n60 = Format Into String(format string=w356, w355) -> (resulting string=w357:string)  [unwired: 2 in, 1 out]
                      }
                      frame "Other" {
                      }
                    }
                    n61 = Format Into String(format string="id_%d_attribute_%d", w272, w269) -> (resulting string=w276:string)  [unwired: 2 in, 1 out]
                    n62 = case shown="\"LabVIEW Class\"" w288 {
                      tunnel: w286 -> [_ w308]
                      tunnel: ["none" ("input 1") w307] -> w270
                      tunnel: w284 -> [_ w306]
                      tunnel: [_ w305] -> w283
                      tunnel: w282 -> [w295 w303]
                      tunnel: [w295 w304] -> w281
                      tunnel: w280 -> [_ w302]
                      tunnel: w279 -> [w294 w301]
                      tunnel: [w294 w300] -> w278
                      tunnel: w276 -> [_ w299]
                      tunnel: w274 -> [_ w298]
                      tunnel: w268 -> [_ w297]
                      frame "UINT8", Default {
                      }
                      frame "LabVIEW Class" {
                        n63 = case shown="Default" w308 {
                          selector: w308 -> [w312 _]
                          tunnel: [w319 "none" ("input 1")] -> w307
                          tunnel: w306 -> [w320 _]
                          tunnel: [w316 ""] -> w305
                          tunnel: [w315 w352] -> w304
                          tunnel: w303 -> [w317 w352]
                          tunnel: w302 -> [w318 _]
                          tunnel: w301 -> [_ w351]
                          tunnel: [w314 w351] -> w300
                          tunnel: w299 -> [w311 _]
                          tunnel: w298 -> [w310 _]
                          tunnel: w297 -> [w309 _]
                          frame Default {
                            n64 = case shown="0, Default" w310 {
                              tunnel: w320 -> [w322 _]
                              tunnel: [w329 "none" ("input 1")] -> w319
                              tunnel: w318 -> [w328 _]
                              tunnel: w317 -> [w327 w350]
                              tunnel: [w326 ""] -> w316
                              tunnel: [w325 w350] -> w315
                              tunnel: w312 -> [w324 _]
                              tunnel: w311 -> [w323 _]
                              tunnel: w309 -> [w321 _]
                              frame 0, Default {
                                n65 = case shown="4, 5" w322 {
                                tunnel: w322 -> [_ w345]
                                tunnel: ["shared" ("input 1") w342] -> w329
                                tunnel: w328 -> [_ w341]
                                tunnel: w327 -> [w331 w340]
                                tunnel: ["" w339] -> w326
                                tunnel: [w331 w338] -> w325
                                tunnel: w324 -> [_ w334]
                                tunnel: w323 -> [_ w335]
                                tunnel: [_ w334] -> _
                                tunnel: w321 -> [_ w333]
                                frame 0, Default {
                                }
                                frame 4, 5 {
                                w344 = T7 5 items=["Depenency", "Inheritance", "Interface Implementation", "Association", "Aggregation", "Composite Aggregation"] ("y")
                                n66 = Equal?(x=w345, y=w344) -> (x = y?=w343:bool)
                                n67 = Select(t="composite", s=w343, f="shared" ("input 1")) -> (s? t:f=w342:string)
                                n68 = Array Size(array=w340) -> (size(s)=w336:i32)
                                n69 = Bundle(w335, w336, w333) -> (w337:cluster{string, i32, i32})  [unwired: 1 out]
                                n70 = Format Into String(format string=w341, w336) -> (resulting string=w339:string)  [unwired: 2 in, 1 out]
                                n71 = Build Array (concatenate)(w340, w337) -> (w338:cluster{string, i32, "index of element":i32}[])
                                }
                                }
                              }
                              frame -1 {
                              }
                            }
                            n72 = Format Into String(format string="type=\"id_class_%d\" " ("input 1"), w312) -> (resulting string=w314:string)  [unwired: 2 in, 1 out]
                          }
                          frame -1 {
                          }
                        }
                      }
                    }
                    n73 = Format Into String(format string=w293, initial string=w275, w272, w269, w271, w270, w278, w283) -> (resulting string=w290:string)  [unwired: 1 in, 1 out]
                  }
                  n74 = Search 1D Array(1D array=w243, element=w249) -> (index of element=w248:i32)  [unwired: 1 out]
                  n75 = for {
                    tunnel: w258 -> [w373] mode=indexing
                    tunnel: w257 -> [w372]
                    tunnel: w239 -> [w367]
                    shift-right: [w369] -> w255
                    shift-left: "" -> [w370]
                    i -> [w366]
                    n76 = call <resource>:"ReversedEngineering_EvaluateMethodText.vi"("String"=w373) -> ("MethodName"=w371:string, "MethodType"=w368:string)  [unwired: 17 out]
                    n77 = Format Into String(format string=w372, initial string=w370, w367, w366, w371, w368) -> (resulting string=w369:string)  [unwired: 1 in, 1 out]
                  }
                  n78 = case shown="-1" w248 {
                    selector: w248 -> [w361 _]
                    tunnel: [w358 _] -> w247
                    tunnel: w246 -> [w362 _]
                    tunnel: w244 -> [w360 _]
                    frame 0, Default {
                      n79 = Index Array(array=w360, index=w361) -> (element=w359:i32)
                      n80 = Format Into String(format string=w362, w359, w359) -> (resulting string=w358:string)  [unwired: 2 in, 1 out]
                    }
                    frame -1 {
                    }
                  }
                  n81 = Concatenate Strings(w253, w255) -> (w254:string)
                  n82 = call <vilib>:"Trim Whitespace.vi"("string"=w254) -> ("trimmed string"=w251:string)  [unwired: 1 in]
                  n83 = Format Into String(format string=w267, initial string=w266, w239, w264, w247, w251) -> (resulting string=w265:string)  [unwired: 1 in, 1 out]
                }
                frame Default {
                }
              }
            }
            n84 = Bundle By Name(cluster=w219, "Text"=w217, "Ass"=w205) -> (w218:T8)
          }
          frame "CreateDataTypes" {
            n85 = Unbundle By Name(w386) -> ("Text"=w380:string, "DataTypes"=w378:T5[])
            n86 = for {
              shift-right: [w388] -> w384
              shift-left: w380 -> [w391]
              tunnel: w387 -> [_]
              tunnel: w383 -> [_]
              tunnel: w382 -> [_]
              tunnel: w379 -> [w390]
              tunnel: w378 -> [w389] mode=indexing
              n87 = Format Into String(format string=w390, initial string=w391, w389, w389) -> (resulting string=w388:string)  [unwired: 1 in, 1 out]
            }
            n88 = call <vilib>:"Trim Whitespace.vi"("string"=w384) -> ("trimmed string"=w377:string)  [unwired: 1 in]
            n89 = Bundle By Name(cluster=w386, "Text"=w377) -> (w385:T8)
          }
          frame "CreateReferedAssociations" {
            n90 = Unbundle By Name(w400) -> ("Text"=w395:string, "Ass"=w394:cluster{string, i32, "index of element":i32}[])
            n91 = for {
              shift-right: [w407] -> w398
              shift-left: w395 -> [w408]
              tunnel: w401 -> [_]
              tunnel: w397 -> [_]
              tunnel: w394 -> [w405] mode=indexing
              # "<ownedMember xmi:type=\"uml:Association\" xmi:id=\"U86ec5265-3719-487c-a13b-3fd45a59c16c\" visibility=\"public\">\n\t\t\t<navigableOwnedEnd xmi:type=\"uml:Property\" xmi:id=\"Uff99e5e3-d87e-49bf-b2a6-6ffcc45f3e01\" name=\"EndName\" visibility=\"protected\" type=\"id_class_0\">\n\t\t\t\t<association xmi:idref=\"U86ec5265-3719-487c-a13b-3fd45a59c16c\"/>\n\t\t\t</navigableOwnedEnd>\n\t\t\t<ownedEnd xmi:type=\"uml:Property\" xmi:id=\"U8ace76fe-f1a0-44ae-9485-5c09a45fdeda\" name=\"StartName\" visibility=\"protected\" type=\"id_class_2\">\n\t\t\t\t<association xmi:idref=\"U86ec5265-3719-487c-a13b-3fd45a59c16c\"/>\n\t\t\t</ownedEnd>\n\t\t\t<ownedEnd xmi:idref=\"Uff99e5e3-d87e-49bf-b2a6-6ffcc45f3e01\"/>\n\t\t\t<memberEnd xmi:idref=\"U8ace76fe-f1a0-44ae-9485-5c09a45fdeda\"/>\n\t\t\t<memberEnd xmi:idref=\"Uff99e5e3-d87e-49bf-b2a6-6ffcc45f3e01\"/>\n\t\t</ownedMember>"
              # "[Some unique ID XYZ]"
              # "[Propertyn/Attributets ID som länkar hit]"
              # "[UNIQUE ID, id_ass_x]"
              n92 = Unbundle(w405) -> (w404:string, w402:i32, "index of element"=w403:i32)
              n93 = Format Into String(format string="\t\t\n<ownedMember xmi:type=\"uml:Association\" xmi:id=\"id_ass_%d\" visibility=\"public\">\n\t\t\t<memberEnd xmi:idref=\"%s\"/>\n\t\t\t<ownedEnd xmi:type=\"uml:Property\" xmi:id=\"id_ass_property_%d\" visibility=\"protected\" type=\"id_class_%d\">\n\t\t\t\t<association xmi:idref=\"id_ass_%d\"/>\n\t\t\t</ownedEnd>\n\t\t\t<memberEnd xmi:idref=\"id_ass_property_%d\"/>\n\t\t</ownedMember>", initial string=w408, w402, w404, w402, w403, w402, w402) -> (resulting string=w407:string)  [unwired: 1 in, 1 out]
            }
            n94 = call <vilib>:"Trim Whitespace.vi"("string"=w398) -> ("trimmed string"=w393:string)  [unwired: 1 in]
            n95 = Bundle By Name(cluster=w400, "Text"=w393) -> (w399:T8)
          }
          frame "CreateNormalAssociations" {
            n96 = Unbundle By Name(w410) -> ("NodeRelationships"=w409:T19)
            n97 = Unbundle By Name(w410) -> ("Text"=w415:string, "Ass"=w412:cluster{string, i32, "index of element":i32}[])
            n98 = Array Size(array=w412) -> (size(s)=w411:i32)
            n99 = for {
              shift-right: [w426] -> w418
              shift-left: w415 -> [w427]
              tunnel: w420 -> [_]
              tunnel: w417 -> [_]
              shift-right: [w425] -> _
              shift-left: w411 -> [w424]
              tunnel: w409 -> [w423] mode=indexing
              i -> [w421]
              n100 = Unbundle(w423) -> (w422:T13)
              n101 = for {
                shift-right: [w434] -> w426
                shift-left: w427 -> [w435]
                shift-right: [w433] -> w425
                shift-left: w424 -> [w432]
                tunnel: w422 -> [w431] mode=indexing
                tunnel: w421 -> [w428]
                (unwired) "\t\t\n<ownedMember xmi:type=\"uml:Association\" xmi:id=\"id_ass_%d\" visibility=\"public\">\n\t\t\t<navigableOwnedEnd xmi:type=\"uml:Property\" xmi:id=\"id_ass_property_%d\" name=\"\" visibility=\"protected\" type=\"id_class_%d\">\n\t\t\t\t<association xmi:idref=\"id_ass_%d\"/>\n\t\t\t</navigableOwnedEnd>\n\t\t\t<ownedEnd xmi:type=\"uml:Property\" xmi:id=\"id_ass_property2_%d\" name=\"\" visibility=\"protected\" type=\"id_class_%d\">\n\t\t\t\t<association xmi:idref=\"id_ass_%d\"/>\n\t\t\t</ownedEnd>\n\t\t\t<ownedEnd xmi:idref=\"id_ass_property_%d\"/>\n\t\t\t<memberEnd xmi:idref=\"id_ass_property2_%d\"/>\n\t\t\t<memberEnd xmi:idref=\"id_ass_property_%d\"/>\n\t\t</ownedMember>"
                (unwired) "\t\t\n<ownedMember xmi:type=\"uml:Association\" xmi:id=\"U86ec5265-3719-487c-a13b-3fd45a59c16c\" visibility=\"public\">\n\t\t\t<navigableOwnedEnd xmi:type=\"uml:Property\" xmi:id=\"Uff99e5e3-d87e-49bf-b2a6-6ffcc45f3e01\" name=\"EndName\" visibility=\"protected\" type=\"id_class_0\">\n\t\t\t\t<association xmi:idref=\"U86ec5265-3719-487c-a13b-3fd45a59c16c\"/>\n\t\t\t</navigableOwnedEnd>\n\t\t\t<ownedEnd xmi:type=\"uml:Property\" xmi:id=\"U8ace76fe-f1a0-44ae-9485-5c09a45fdeda\" name=\"StartName\" visibility=\"protected\" type=\"id_class_2\">\n\t\t\t\t<association xmi:idref=\"U86ec5265-3719-487c-a13b-3fd45a59c16c\"/>\n\t\t\t</ownedEnd>\n\t\t\t<ownedEnd xmi:idref=\"Uff99e5e3-d87e-49bf-b2a6-6ffcc45f3e01\"/>\n\t\t\t<memberEnd xmi:idref=\"U8ace76fe-f1a0-44ae-9485-5c09a45fdeda\"/>\n\t\t\t<memberEnd xmi:idref=\"Uff99e5e3-d87e-49bf-b2a6-6ffcc45f3e01\"/>\n\t\t</ownedMember>"
                (unwired) "\t\t\n<ownedMember xmi:type=\"uml:Association\" xmi:id=\"id_ass_%d\" visibility=\"public\">\n\t\t\t<memberEnd xmi:idref=\"%s\"/>\n\t\t\t<ownedEnd xmi:type=\"uml:Property\" xmi:id=\"id_ass_property_%d\" visibility=\"protected\" type=\"id_class_%d\">\n\t\t\t\t<association xmi:idref=\"id_ass_%d\"/>\n\t\t\t</ownedEnd>\n\t\t\t<memberEnd xmi:idref=\"id_ass_property_%d\"/>\n\t\t</ownedMember>"
                n102 = Unbundle By Name(w431) -> ("RelationType"=w430:T7, "index of element"=w429:i32)
                n103 = case shown="0" w430 {
                  tunnel: w435 -> [w436 w444 w451]
                  tunnel: [w436 w443 w450] -> w434
                  tunnel: [w437 w442 w449] -> w433
                  tunnel: w432 -> [w437 w439 w445]
                  tunnel: w429 -> [_ w438 w446]
                  tunnel: w428 -> [_ w441 w447]
                  frame Default {
                  }
                  frame 3 {
                    (unwired) T7 3 items=["Depenency", "Inheritance", "Interface Implementation", "Association", "Aggregation", "Composite Aggregation"] ("element")
                    n104 = Format Into String(format string="\t\t\n<ownedMember xmi:type=\"uml:Association\" xmi:id=\"id_ass_%d\" visibility=\"public\">\n\t\t\t<navigableOwnedEnd xmi:type=\"uml:Property\" xmi:id=\"id_ass_property_%d\" name=\"\" visibility=\"protected\" type=\"id_class_%d\">\n\t\t\t\t<association xmi:idref=\"id_ass_%d\"/>\n\t\t\t</navigableOwnedEnd>\n\t\t\t<ownedEnd xmi:type=\"uml:Property\" xmi:id=\"id_ass_property2_%d\" name=\"\" visibility=\"protected\" type=\"id_class_%d\">\n\t\t\t\t<association xmi:idref=\"id_ass_%d\"/>\n\t\t\t</ownedEnd>\n\t\t\t<ownedEnd xmi:idref=\"id_ass_property_%d\"/>\n\t\t\t<memberEnd xmi:idref=\"id_ass_property2_%d\"/>\n\t\t\t<memberEnd xmi:idref=\"id_ass_property_%d\"/>\n\t\t</ownedMember>", initial string=w444, w439, w439, w438, w439, w439, w441, w439, w439, w439, w439) -> (resulting string=w443:string)  [unwired: 1 in, 1 out]
                    n105 = Increment(x=w439) -> (x+1=w442:i32)
                  }
                  frame 0 {
                    (unwired) T7 3 items=["Depenency", "Inheritance", "Interface Implementation", "Association", "Aggregation", "Composite Aggregation"] ("element")
                    n106 = Format Into String(format string="\t\t\n<packagedElement xmi:type=\"uml:Dependency\" xmi:id=\"id_dep_%d\" visibility=\"public\" supplier=\"id_class_%d\" client=\"id_class_%d\" /> ", initial string=w451, w445, w446, w447) -> (resulting string=w450:string)  [unwired: 1 in, 1 out]
                    n107 = Increment(x=w445) -> (x+1=w449:i32)
                  }
                }
              }
            }
            n108 = call <vilib>:"Trim Whitespace.vi"("string"=w418) -> ("trimmed string"=w414:string)  [unwired: 1 in]
            n109 = Bundle By Name(cluster=w410, "Text"=w414) -> (w419:T8)
          }
        }
        n110 = Equal?(x=w58, y="Exit") -> (x = y?=w60:bool)
        n111 = Select(t="Error", s=w57, f=w58) -> (s? t:f=w61:string)
      }
      n112 = Unbundle By Name(w19) -> ("Text"=w18:string)
    }
    frame Error {
    }
  }
  "reference out" <- w12
  "error out" <- w13
  "XMIText" <- w3
